vi "SV Cells.vi"(3 "error in":errorcluster, 4 "End 2":cluster{"Column":i32, "Row":i32}={"Column"=1, "Row"=2}, 5 "Refnum Cluster In":T1, 6 "Start 2":cluster{"Column":i32, "Row":i32}={"Column"=1, "Row"=1}) -> (0 "Error Out":errorcluster, 1 "Refnum Cluster Out":T1, 2 "Data":string[][](array[string]))   [LabVIEW 2010]
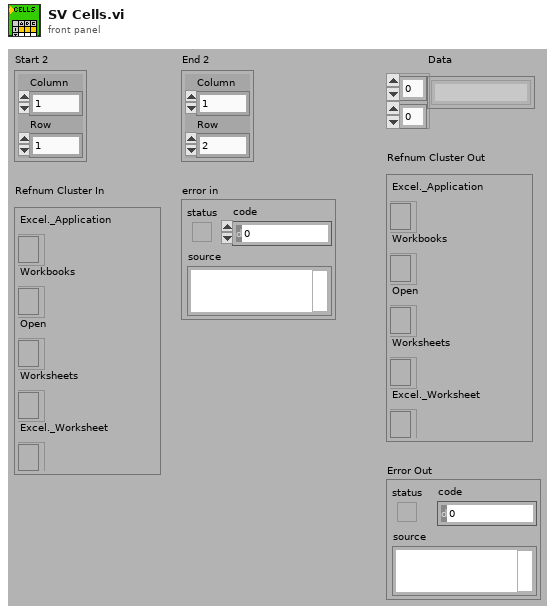
[diagram p1: front panel]
types:
  T1 = cluster{"Excel._Application":refnum<k7>, "Workbooks":refnum<k7>, "Open":refnum<k7>, "Worksheets":refnum<k7>, "Excel._Worksheet":refnum<k7>}
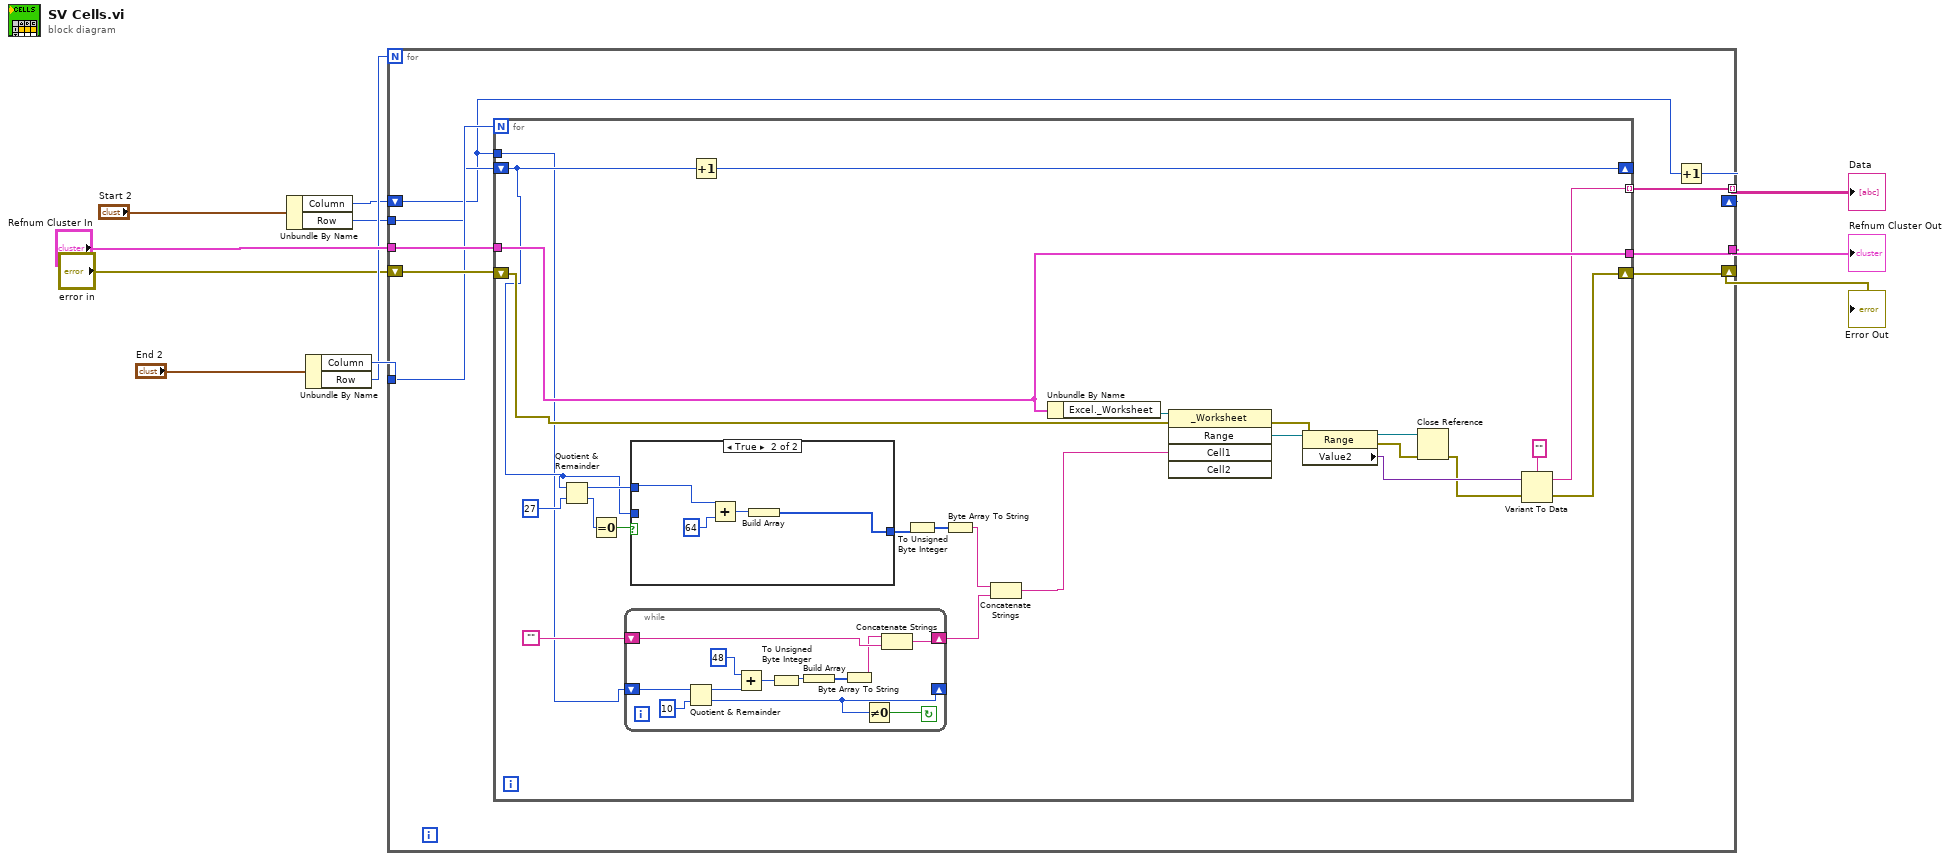
[diagram p0: block diagram]
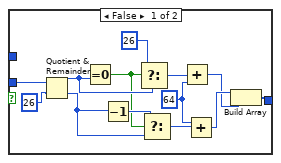
[diagram p2: hidden frame]
diagram:
  n1 = Unbundle By Name("Start 2") -> ("Column"=w3:i32, "Row"=w2:i32)
  n2 = Unbundle By Name("End 2") -> ("Column"=w5:i32, "Row"=w4:i32)
  n3 = for {
    N: w4 -> [_]
    tunnel: "Refnum Cluster In" -> [w20]
    tunnel: [w18] -> w7
    shift-right: [w17] -> w8
    shift-left: "error in" -> [w19]
    tunnel: w5 -> [w16]
    tunnel: w2 -> [w15]
    tunnel: [w14] -> w6 mode=indexing
    shift-right: [w13] -> _
    shift-left: w3 -> [w12]
    n4 = for {
      N: w16 -> [_]
      tunnel: w20 -> [w25]
      tunnel: [w25] -> w18
      shift-right: [w23] -> w17
      shift-left: w19 -> [w26]
      tunnel: w12 -> [w21]
      tunnel: [w24] -> w14 mode=indexing
      shift-right: [w45] -> _
      shift-left: w15 -> [w22]
      n5 = Quotient & Remainder(x=w22, y=27) -> (x-y*floor(x/y)=w33:i32, floor(x/y)=w34:i32)
      n6 = Equal To 0?(x=w34) -> (x = 0?=w35:bool)
      n7 = while {
        shift-left: w21 -> [w57]
        shift-right: [w48] -> _
        shift-left: "" -> [w47]
        shift-right: [w50] -> w28
        stop <- w49 continue-if-true
        n8 = Quotient & Remainder(x=w57, y=10) -> (x-y*floor(x/y)=w55:i32, floor(x/y)=w48:i32)
        n9 = Add(x=48, y=w55) -> (x+y=w53:i32)
        n10 = To Unsigned Byte Integer(number=w53) -> (unsigned 8bit integer=w52:u8)
        n11 = Build Array(w52) -> (w51:u8[])
        n12 = Byte Array To String(unsigned byte array=w51) -> (string=w46:string)
        n13 = Not Equal To 0?(x=w48) -> (x != 0?=w49:bool)
        n14 = Concatenate Strings(w46, w47) -> (w50:string)
      }
      n15 = case shown="True" w35 {
        tunnel: w22 -> [w70 _]
        tunnel: w33 -> [_ w74]
        tunnel: [w59 w73] -> w32
        frame False {
          w58 = 64
          n16 = Quotient & Remainder(x=w70, y=26) -> (x-y*floor(x/y)=w67:i32, floor(x/y)=w64:i32)
          n17 = Equal To 0?(x=w67) -> (x = 0?=w65:bool)
          n18 = Decrement(x=w64) -> (x-1=w66:i32)
          n19 = Select(t=26, s=w65, f=w67) -> (s? t:f=w63:i32)
          n20 = Select(t=w66, s=w65, f=w64) -> (s? t:f=w62:i32)
          n21 = Add(x=w63, y=w58) -> (x+y=w60:i32)
          n22 = Add(x=w58, y=w62) -> (x+y=w61:i32)
          n23 = Build Array(w61, w60) -> (w59:i32[])
        }
        frame True {
          n24 = Add(x=w74, y=64) -> (x+y=w71:i32)
          n25 = Build Array(w71) -> (w73:i32[])
        }
      }
      n26 = Increment(x=w22) -> (x+1=w45:i32)
      n27 = To Unsigned Byte Integer(number=w32) -> (unsigned 8bit integer=w31:u8[])
      n28 = Byte Array To String(unsigned byte array=w31) -> (string=w29:string)
      n29 = Concatenate Strings(w29, w28) -> (w27:string)
      n30 = Unbundle By Name(w25) -> ("Excel._Worksheet"=w37:refnum<k7>)
      n31 = invoke class="_Worksheet" method="Range"(reference=w37, error in=w26, "Cell1"=w27) -> (error out=w44:errorcluster, "Range"=w43:refnum<k7>)  [unwired: 2 in, 3 out]
      n32 = property class="Range"(reference=w43, error in=w44) -> (reference out=w42:refnum<k7>, error out=w41:errorcluster, "Value2"=w40:variant)
      n33 = Close Reference(reference=w42, error in (no error)=w41) -> (error out=w39:errorcluster)
      n34 = Variant To Data(error in=w39, Variant=w40, type="") -> (error out=w23:errorcluster, data=w24:string)
    }
    n35 = Increment(x=w12) -> (x+1=w13:i32)
  }
  "Data" <- w6
  "Refnum Cluster Out" <- w7
  "Error Out" <- w8
